vi "ploter.vi"() -> ()   [LabVIEW 2011]
panel:
  in  "SLM 1":bool
  in  "T --> A":bool
  in  "Boolean":bool
  in  "stop":bool
  in  "Quarter Wave Plate":dbl
  in  "Half Wave Plate":dbl
  out "Amplitude":T1(plugin-control)
  out "Phase":T1(plugin-control)
  out "Polar":T1(plugin-control)
  # "SLM 2"
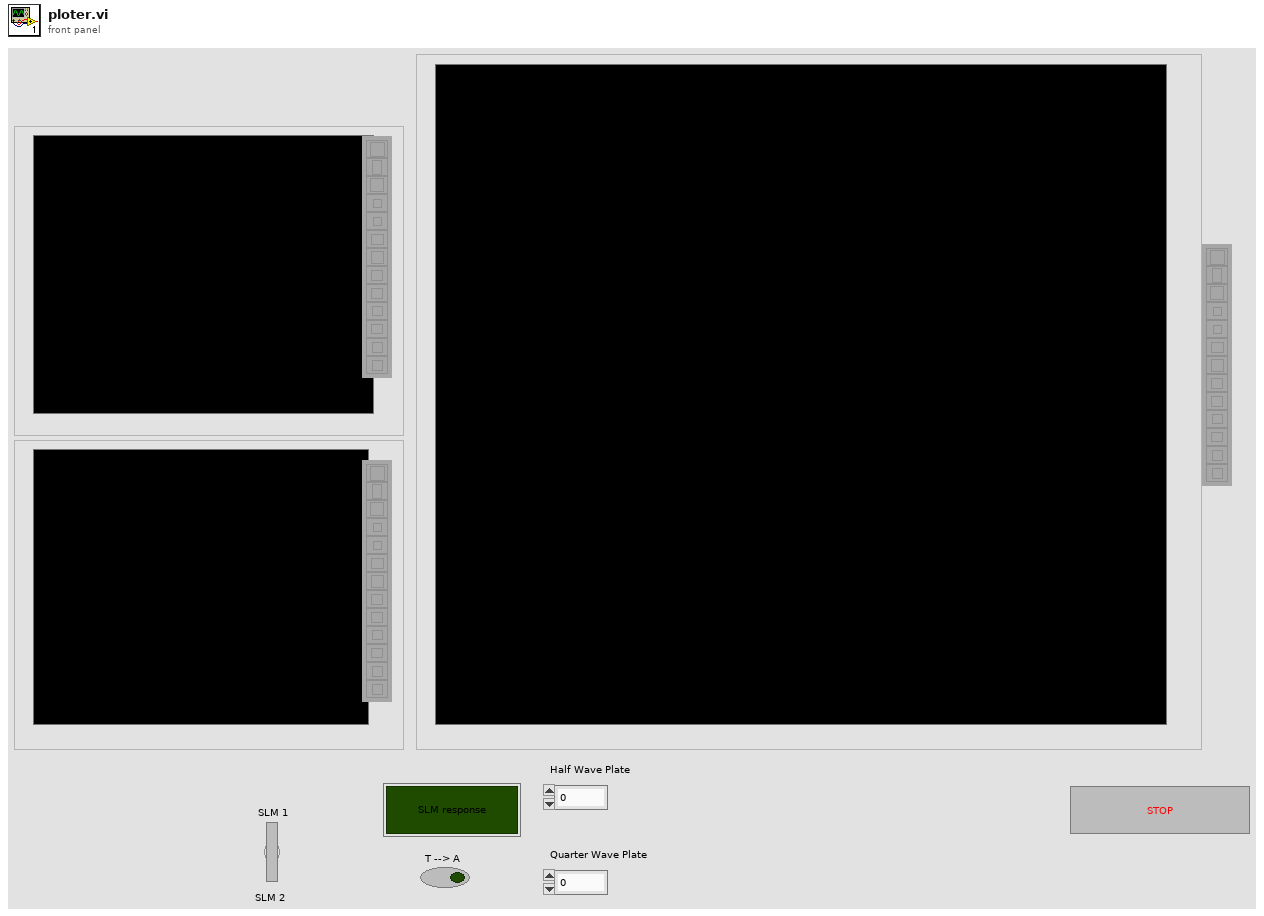
[diagram p1: front panel]
types:
  T1 = typedef "IMAQ Image.ctl" = refnum<image>
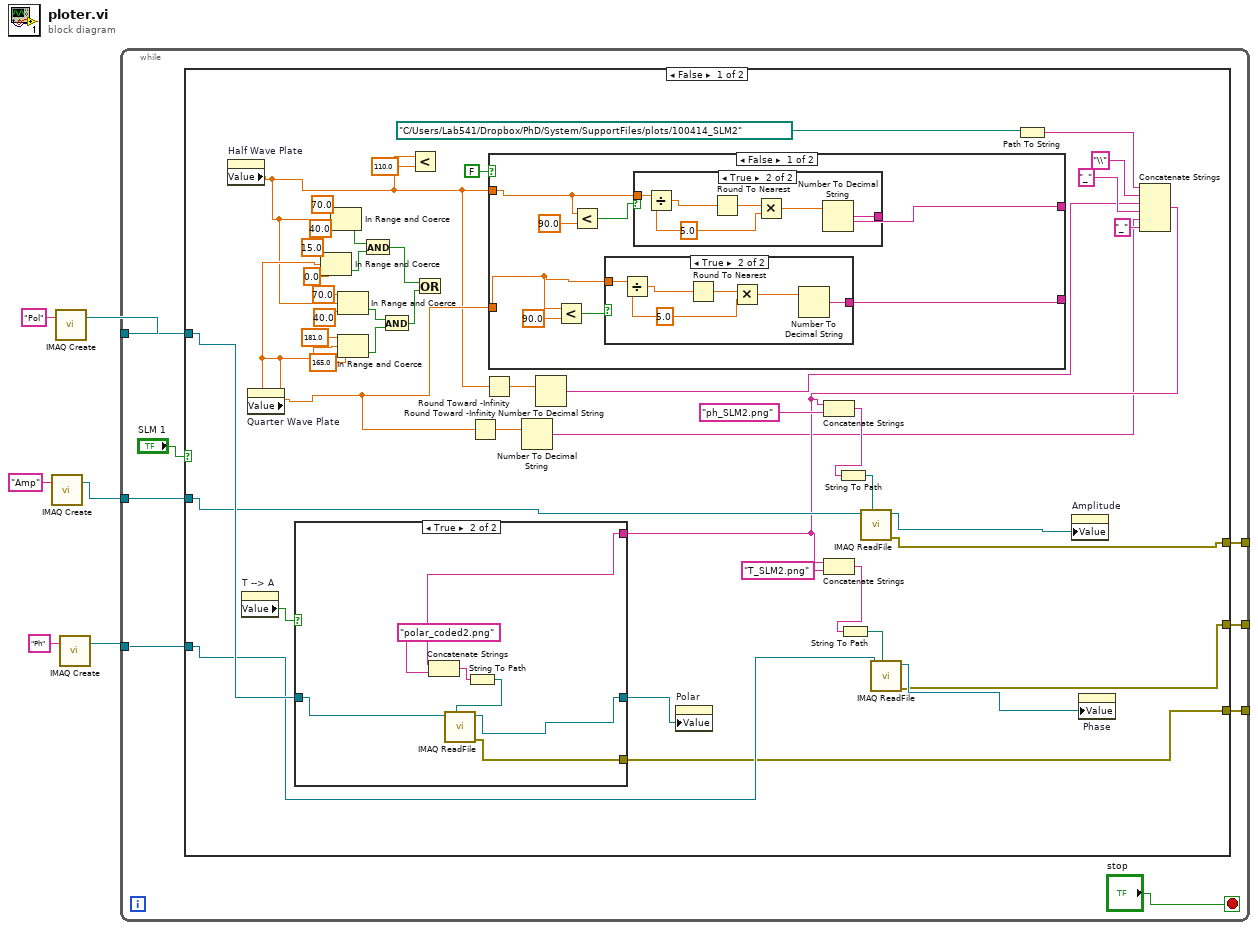
[diagram p0: block diagram]
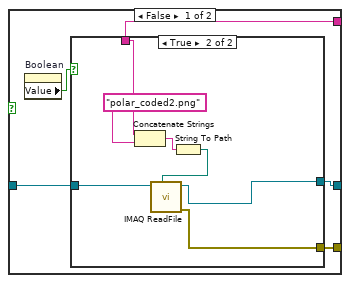
[diagram p2: hidden frame]
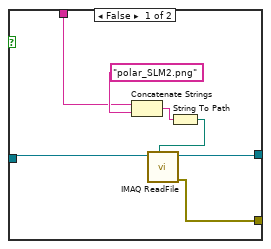
[diagram p3: hidden frame]
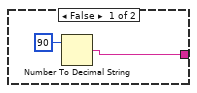
[diagram p4: hidden frame]
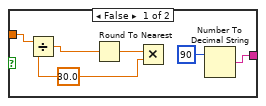
[diagram p5: hidden frame]
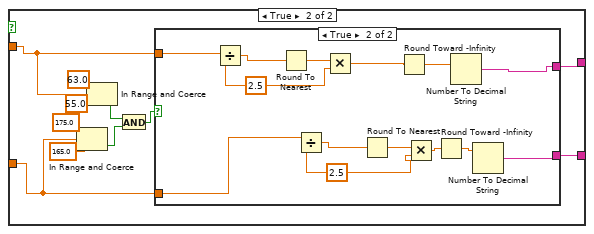
[diagram p6: hidden frame]
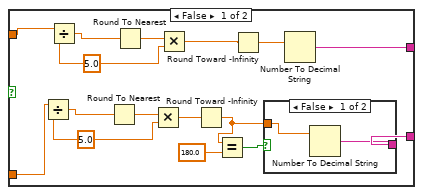
[diagram p7: hidden frame]
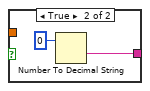
[diagram p8: hidden frame]
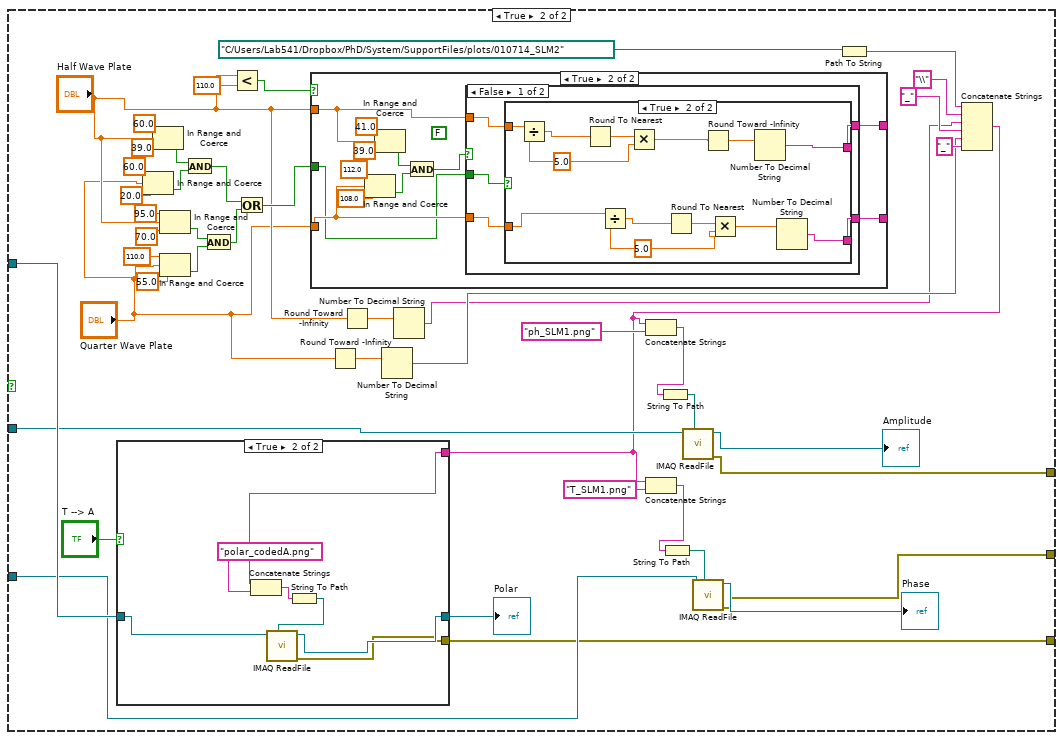
[diagram p9: hidden frame]
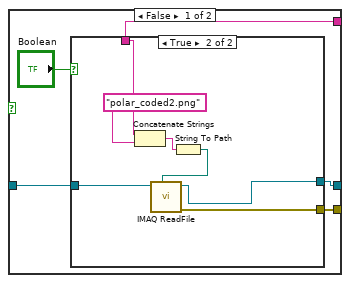
[diagram p10: hidden frame]
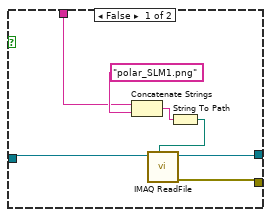
[diagram p11: hidden frame]
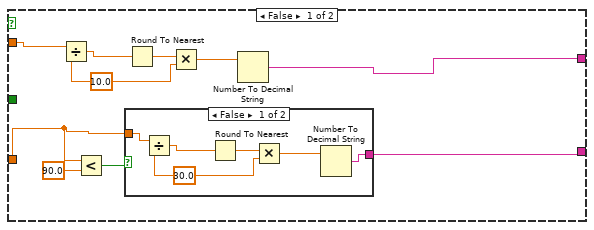
[diagram p12: hidden frame]
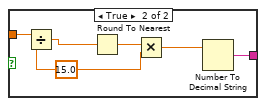
[diagram p13: hidden frame]
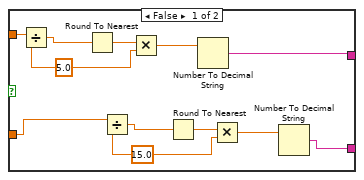
[diagram p14: hidden frame]
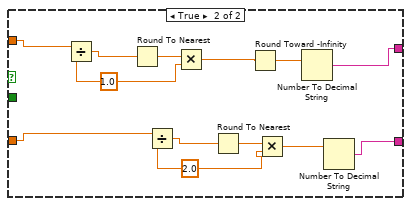
[diagram p15: hidden frame]
diagram:
  n1 = call "IMAQ Create"("Image Name"="Amp") -> ("New Image"=w5:T1)  [unwired: 4 in, 1 out]
  n2 = call "IMAQ Create"("Image Name"="Pol") -> ("New Image"=w6:T1)  [unwired: 4 in, 1 out]
  n3 = call "IMAQ Create"("Image Name"="Ph") -> ("New Image"=w4:T1)  [unwired: 4 in, 1 out]
  n4 = while {
    tunnel: w6 -> [w14]
    tunnel: w5 -> [w13]
    tunnel: w4 -> [w12]
    tunnel: [w9] -> _
    tunnel: [w8] -> _
    tunnel: [w7] -> _
    stop <- "stop" stop-if-true
    n5 = case shown="False" "SLM 1" {
      tunnel: w14 -> [w58 w202]
      tunnel: w13 -> [w57 w201]
      tunnel: w12 -> [w56 w200]
      tunnel: [w21 w166] -> w9
      tunnel: [w22 w165] -> w8
      tunnel: [w23 w164] -> w7
      frame False {
        n6 = property on="Half Wave Plate" class="DigNum (strict)"() -> ("Value"=w17:dbl)  [unwired: 2 in, 2 out]
        n7 = property on="T --> A" class="Bool (strict)"() -> ("Value"=w26:bool)  [unwired: 2 in, 2 out]
        n8 = property on="Quarter Wave Plate" class="DigNum (strict)"() -> ("Value"=w18:dbl)  [unwired: 2 in, 2 out]
        n9 = In Range and Coerce(upper limit=15.0, x=w18, lower limit=0.0) -> (In Range?=w38:bool)  [unwired: 1 out]
        n10 = In Range and Coerce(upper limit=70.0, x=w17, lower limit=40.0) -> (In Range?=w39:bool)  [unwired: 1 out]
        n11 = In Range and Coerce(upper limit=70.0, x=w17, lower limit=40.0) -> (In Range?=w37:bool)  [unwired: 1 out]
        n12 = In Range and Coerce(upper limit=181.0, x=w18, lower limit=165.0) -> (In Range?=w36:bool)  [unwired: 1 out]
        n13 = And(x=w39, y=w38) -> (x .and. y?=w35:bool)
        n14 = And(x=w37, y=w36) -> (x .and. y?=w25:bool)
        n15 = Less?(x=w17, y=110.0) -> ()  [unwired: 1 out]
        n16 = Or(x=w35, y=w25) -> ()  [unwired: 1 out]
        n17 = Round Toward -Infinity(1:w18) -> (0:w19:dbl)
        n18 = Round Toward -Infinity(1:w17) -> (0:w20:dbl)
        n19 = case shown="False" FALSE {
          tunnel: [w92 w123] -> _
          tunnel: [w91 w122] -> _
          tunnel: w18 -> [w90 w114]
          tunnel: w17 -> [w87 w115]
          frame False {
            n20 = Less?(x=w90, y=90.0) -> (x < y?=w88:bool)
            n21 = Less?(x=w87, y=90.0) -> (x < y?=w85:bool)
            n22 = case shown="True" w88 {
              tunnel: w90 -> [w104 w109]
              tunnel: [w103 w108] -> w91
              frame False {
                w102 = 30.0 ("y")
                n23 = Divide(x=w104, y=w102) -> (x/y=w106:dbl)
                n24 = Round To Nearest(number=w106) -> (nearest integer value=w105:dbl)
                n25 = Multiply(x=w105, y=w102) -> ()  [unwired: 1 out]
                n26 = Number To Decimal String(number=90) -> (decimal integer string=w103:string)  [unwired: 1 in]
              }
              frame True {
                w107 = 5.0 ("y")
                n27 = Divide(x=w109, y=w107) -> (x/y=w112:dbl)
                n28 = Round To Nearest(number=w112) -> (nearest integer value=w111:dbl)
                n29 = Multiply(x=w111, y=w107) -> (x*y=w110:dbl)
                n30 = Number To Decimal String(number=w110) -> (decimal integer string=w108:string)  [unwired: 1 in]
              }
            }
            n31 = case shown="True" w85 {
              tunnel: w87 -> [_ w97]
              tunnel: [w94 w96] -> w92
              frame False {
                n32 = Number To Decimal String(number=90) -> (decimal integer string=w94:string)  [unwired: 1 in]
              }
              frame True {
                w95 = 5.0 ("y")
                n33 = Divide(x=w97, y=w95) -> (x/y=w100:dbl)
                n34 = Round To Nearest(number=w100) -> (nearest integer value=w99:dbl)
                n35 = Multiply(x=w99, y=w95) -> (x*y=w98:dbl)
                n36 = Number To Decimal String(number=w98) -> (decimal integer string=w96:string)  [unwired: 1 in]
              }
            }
          }
          frame True {
            n37 = In Range and Coerce(upper limit=175.0, x=w114, lower limit=165.0) -> (In Range?=w116:bool)  [unwired: 1 out]
            n38 = In Range and Coerce(upper limit=63.0, x=w115, lower limit=55.0) -> (In Range?=w117:bool)  [unwired: 1 out]
            n39 = And(x=w117, y=w116) -> (x .and. y?=w113:bool)
            n40 = case shown="True" w113 {
              tunnel: [w130 w147] -> w123
              tunnel: [w129 w146] -> w122
              tunnel: w115 -> [w125 w149]
              tunnel: w114 -> [w124 w148]
              frame False {
                w131 = 5.0 ("y")
                w135 = 5.0 ("y")
                n41 = Divide(x=w124, y=w131) -> (x/y=w134:dbl)
                n42 = Divide(x=w125, y=w135) -> (x/y=w139:dbl)
                n43 = Round To Nearest(number=w134) -> (nearest integer value=w133:dbl)
                n44 = Round To Nearest(number=w139) -> (nearest integer value=w138:dbl)
                n45 = Multiply(x=w133, y=w131) -> (x*y=w132:dbl)
                n46 = Multiply(x=w138, y=w135) -> (x*y=w137:dbl)
                n47 = Round Toward -Infinity(1:w132) -> (0:w128:dbl)
                n48 = Equal?(x=w128, y=180.0) -> (x = y?=w126:bool)
                n49 = Round Toward -Infinity(1:w137) -> (0:w136:dbl)
                n50 = case shown="False" w126 {
                  tunnel: [w140 w143] -> w129
                  tunnel: w128 -> [w141 _]
                  frame False {
                    n51 = Number To Decimal String(number=w141) -> (decimal integer string=w140:string)  [unwired: 1 in]
                  }
                  frame True {
                    n52 = Number To Decimal String(number=0) -> (decimal integer string=w143:string)  [unwired: 1 in]
                  }
                }
                n53 = Number To Decimal String(number=w136) -> (decimal integer string=w130:string)  [unwired: 1 in]
              }
              frame True {
                w150 = 2.5 ("y")
                w151 = 2.5 ("y")
                n54 = Divide(x=w149, y=w151) -> (x/y=w157:dbl)
                n55 = Round To Nearest(number=w157) -> (nearest integer value=w156:dbl)
                n56 = Divide(x=w148, y=w150) -> (x/y=w155:dbl)
                n57 = Multiply(x=w156, y=w151) -> (x*y=w153:dbl)
                n58 = Round To Nearest(number=w155) -> (nearest integer value=w154:dbl)
                n59 = Round Toward -Infinity(1:w153) -> (0:w152:dbl)
                n60 = Multiply(x=w154, y=w150) -> (x*y=w145:dbl)
                n61 = Round Toward -Infinity(1:w145) -> (0:w144:dbl)
                n62 = Number To Decimal String(number=w152) -> (decimal integer string=w147:string)  [unwired: 1 in]
                n63 = Number To Decimal String(number=w144) -> (decimal integer string=w146:string)  [unwired: 1 in]
              }
            }
          }
        }
        n64 = Number To Decimal String(number=w19) -> (decimal integer string=w15:string)  [unwired: 1 in]
        n65 = Number To Decimal String(number=w20) -> (decimal integer string=w16:string)  [unwired: 1 in]
        n66 = Path To String(path=path "C:/Users/Lab541/Dropbox/PhD/System/SupportFiles/plots/100414_SLM2" ("File Path")) -> (string=w52:string)
        n67 = Concatenate Strings(w52, "\\" ("string"), w16, "_" ("string"), w15, "_" ("string")) -> (w41:string)
        n68 = case shown="True" w26 {
          tunnel: w58 -> [w63 w79]
          tunnel: [w62 w80] -> w27
          tunnel: w41 -> [w61 w81]
          tunnel: [w59 w78] -> w21
          frame False {
            n69 = property on="Boolean" class="Bool (strict)"() -> ("Value"=w60:bool)  [unwired: 2 in, 2 out]
            n70 = case shown="True" w60 {
              tunnel: w63 -> [w67 w77]
              tunnel: w61 -> [w65 w73]
              tunnel: [w66 w72] -> w62
              tunnel: [w64 w71] -> w59
              frame False {
                n71 = Concatenate Strings(w65, "polar_SLM2.png" ("string")) -> (w69:string)
                n72 = String To Path(string=w69) -> (path=w68:path)
                n73 = call "IMAQ ReadFile"("File Path"=w68, "Image"=w67) -> ("error out"=w64:errorcluster, "Image Out"=w66:T1)  [unwired: 5 in, 3 out]
              }
              frame True {
                n74 = Concatenate Strings(w73, "polar_coded2.png" ("string")) -> (w75:string)
                n75 = String To Path(string=w75) -> (path=w74:path)
                n76 = call "IMAQ ReadFile"("File Path"=w74, "Image"=w77) -> ("error out"=w71:errorcluster, "Image Out"=w72:T1)  [unwired: 5 in, 3 out]
              }
            }
          }
          frame True {
            n77 = Concatenate Strings(w81, "polar_coded2.png" ("string")) -> (w83:string)
            n78 = String To Path(string=w83) -> (path=w82:path)
            n79 = call "IMAQ ReadFile"("File Path"=w82, "Image"=w79) -> ("error out"=w78:errorcluster, "Image Out"=w80:T1)  [unwired: 5 in, 3 out]
          }
        }
        n80 = property on="Polar" class="ImageControl"("Value"=w27) -> ()  [unwired: 2 in, 2 out]
        n81 = Concatenate Strings(w41, "ph_SLM2.png" ("string")) -> (w49:string)
        n82 = Concatenate Strings(w41, "T_SLM2.png" ("string")) -> (w46:string)
        n83 = String To Path(string=w49) -> (path=w48:path)
        n84 = String To Path(string=w46) -> (path=w45:path)
        n85 = call "IMAQ ReadFile"("File Path"=w48, "Image"=w57) -> ("error out"=w23:errorcluster, "Image Out"=w29:T1)  [unwired: 5 in, 3 out]
        n86 = call "IMAQ ReadFile"("File Path"=w45, "Image"=w56) -> ("error out"=w22:errorcluster, "Image Out"=w28:T1)  [unwired: 5 in, 3 out]
        n87 = property on="Amplitude" class="ImageControl"("Value"=w29) -> ()  [unwired: 2 in, 2 out]
        n88 = property on="Phase" class="ImageControl"("Value"=w28) -> ()  [unwired: 2 in, 2 out]
      }
      frame True {
        n89 = In Range and Coerce(upper limit=60.0, x="Quarter Wave Plate", lower limit=20.0) -> (In Range?=w179:bool)  [unwired: 1 out]
        n90 = In Range and Coerce(upper limit=60.0, x="Half Wave Plate", lower limit=39.0) -> (In Range?=w180:bool)  [unwired: 1 out]
        n91 = In Range and Coerce(upper limit=95.0, x="Half Wave Plate", lower limit=70.0) -> (In Range?=w178:bool)  [unwired: 1 out]
        n92 = In Range and Coerce(upper limit=110.0, x="Quarter Wave Plate", lower limit=55.0) -> (In Range?=w177:bool)  [unwired: 1 out]
        n93 = And(x=w180, y=w179) -> (x .and. y?=w175:bool)
        n94 = And(x=w178, y=w177) -> (x .and. y?=w176:bool)
        n95 = Less?(x="Half Wave Plate", y=110.0) -> (x < y?=w168:bool)
        n96 = Or(x=w175, y=w176) -> (x .or. y?=w174:bool)
        n97 = case shown="True" w168 {
          tunnel: [w234 w262] -> _
          tunnel: [w233 w261] -> _
          tunnel: w174 -> [_ w252]
          tunnel: "Quarter Wave Plate" -> [w232 w253]
          tunnel: "Half Wave Plate" -> [w235 w254]
          frame False {
            w229 = 10.0 ("y")
            n98 = Divide(x=w235, y=w229) -> (x/y=w238:dbl)
            n99 = Less?(x=w232, y=90.0) -> (x < y?=w230:bool)
            n100 = case shown="False" w230 {
              tunnel: w232 -> [w241 w247]
              tunnel: [w240 w246] -> w233
              frame False {
                w239 = 30.0 ("y")
                n101 = Divide(x=w241, y=w239) -> (x/y=w244:dbl)
                n102 = Round To Nearest(number=w244) -> (nearest integer value=w243:dbl)
                n103 = Multiply(x=w243, y=w239) -> (x*y=w242:dbl)
                n104 = Number To Decimal String(number=w242) -> (decimal integer string=w240:string)  [unwired: 1 in]
              }
              frame True {
                w245 = 15.0 ("y")
                n105 = Divide(x=w247, y=w245) -> (x/y=w250:dbl)
                n106 = Round To Nearest(number=w250) -> (nearest integer value=w249:dbl)
                n107 = Multiply(x=w249, y=w245) -> (x*y=w248:dbl)
                n108 = Number To Decimal String(number=w248) -> (decimal integer string=w246:string)  [unwired: 1 in]
              }
            }
            n109 = Round To Nearest(number=w238) -> (nearest integer value=w237:dbl)
            n110 = Multiply(x=w237, y=w229) -> (x*y=w236:dbl)
            n111 = Number To Decimal String(number=w236) -> (decimal integer string=w234:string)  [unwired: 1 in]
          }
          frame True {
            (unwired) FALSE
            n112 = In Range and Coerce(upper limit=112.0, x=w253, lower limit=108.0) -> (In Range?=w255:bool)  [unwired: 1 out]
            n113 = In Range and Coerce(upper limit=41.0, x=w254, lower limit=39.0) -> (In Range?=w256:bool)  [unwired: 1 out]
            n114 = And(x=w256, y=w255) -> (x .and. y?=w251:bool)
            n115 = case shown="False" w251 {
              tunnel: [w267 w294] -> w262
              tunnel: [w266 w293] -> w261
              tunnel: w252 -> [w265 _]
              tunnel: w253 -> [w264 w295]
              tunnel: w254 -> [w263 w296]
              frame False {
                n116 = case shown="True" w265 {
                  tunnel: [w271 w292] -> w267
                  tunnel: [w270 w291] -> w266
                  tunnel: w264 -> [w273 w290]
                  tunnel: w263 -> [w272 w289]
                  frame False {
                    w268 = 15.0 ("y")
                    w269 = 5.0 ("y")
                    n117 = Divide(x=w272, y=w269) -> (x/y=w279:dbl)
                    n118 = Round To Nearest(number=w279) -> (nearest integer value=w278:dbl)
                    n119 = Divide(x=w273, y=w268) -> (x/y=w276:dbl)
                    n120 = Multiply(x=w278, y=w269) -> (x*y=w277:dbl)
                    n121 = Round To Nearest(number=w276) -> (nearest integer value=w275:dbl)
                    n122 = Number To Decimal String(number=w277) -> (decimal integer string=w271:string)  [unwired: 1 in]
                    n123 = Multiply(x=w275, y=w268) -> (x*y=w274:dbl)
                    n124 = Number To Decimal String(number=w274) -> (decimal integer string=w270:string)  [unwired: 1 in]
                  }
                  frame True {
                    w280 = 5.0 ("y")
                    w281 = 5.0 ("y")
                    n125 = Divide(x=w289, y=w281) -> (x/y=w288:dbl)
                    n126 = Round To Nearest(number=w288) -> (nearest integer value=w287:dbl)
                    n127 = Divide(x=w290, y=w280) -> (x/y=w286:dbl)
                    n128 = Multiply(x=w287, y=w281) -> (x*y=w283:dbl)
                    n129 = Round To Nearest(number=w286) -> (nearest integer value=w285:dbl)
                    n130 = Round Toward -Infinity(1:w283) -> (0:w282:dbl)
                    n131 = Multiply(x=w285, y=w280) -> (x*y=w284:dbl)
                    n132 = Number To Decimal String(number=w282) -> (decimal integer string=w292:string)  [unwired: 1 in]
                    n133 = Number To Decimal String(number=w284) -> (decimal integer string=w291:string)  [unwired: 1 in]
                  }
                }
              }
              frame True {
                w297 = 2.0 ("y")
                w298 = 1.0 ("y")
                n134 = Divide(x=w296, y=w298) -> (x/y=w305:dbl)
                n135 = Round To Nearest(number=w305) -> (nearest integer value=w304:dbl)
                n136 = Divide(x=w295, y=w297) -> (x/y=w303:dbl)
                n137 = Multiply(x=w304, y=w298) -> (x*y=w300:dbl)
                n138 = Round To Nearest(number=w303) -> (nearest integer value=w302:dbl)
                n139 = Round Toward -Infinity(1:w300) -> (0:w299:dbl)
                n140 = Multiply(x=w302, y=w297) -> (x*y=w301:dbl)
                n141 = Number To Decimal String(number=w299) -> (decimal integer string=w294:string)  [unwired: 1 in]
                n142 = Number To Decimal String(number=w301) -> (decimal integer string=w293:string)  [unwired: 1 in]
              }
            }
          }
        }
        n143 = Round Toward -Infinity(1:"Quarter Wave Plate") -> (0:w160:dbl)
        n144 = Round Toward -Infinity(1:"Half Wave Plate") -> (0:w161:dbl)
        n145 = Number To Decimal String(number=w160) -> (decimal integer string=w159:string)  [unwired: 1 in]
        n146 = Number To Decimal String(number=w161) -> (decimal integer string=w158:string)  [unwired: 1 in]
        n147 = Path To String(path=path "C:/Users/Lab541/Dropbox/PhD/System/SupportFiles/plots/010714_SLM2" ("File Path")) -> (string=w194:string)
        n148 = Concatenate Strings(w194, "\\" ("string"), w158, "_" ("string"), w159, "_" ("string")) -> (w182:string)
        n149 = case shown="True" "T --> A" {
          tunnel: w202 -> [w207 w223]
          tunnel: [w205 w224] -> w183
          tunnel: w182 -> [w204 w225]
          tunnel: [w203 w222] -> w166
          frame False {
            n150 = case shown="True" "Boolean" {
              tunnel: w207 -> [w211 w221]
              tunnel: w204 -> [w209 w217]
              tunnel: [w210 w216] -> w205
              tunnel: [w208 w215] -> w203
              frame False {
                n151 = Concatenate Strings(w209, "polar_SLM1.png" ("string")) -> (w213:string)
                n152 = String To Path(string=w213) -> (path=w212:path)
                n153 = call "IMAQ ReadFile"("File Path"=w212, "Image"=w211) -> ("error out"=w208:errorcluster, "Image Out"=w210:T1)  [unwired: 5 in, 3 out]
              }
              frame True {
                n154 = Concatenate Strings(w217, "polar_coded2.png" ("string")) -> (w219:string)
                n155 = String To Path(string=w219) -> (path=w218:path)
                n156 = call "IMAQ ReadFile"("File Path"=w218, "Image"=w221) -> ("error out"=w215:errorcluster, "Image Out"=w216:T1)  [unwired: 5 in, 3 out]
              }
            }
          }
          frame True {
            n157 = Concatenate Strings(w225, "polar_codedA.png" ("string")) -> (w227:string)
            n158 = String To Path(string=w227) -> (path=w226:path)
            n159 = call "IMAQ ReadFile"("File Path"=w226, "Image"=w223) -> ("error out"=w222:errorcluster, "Image Out"=w224:T1)  [unwired: 5 in, 3 out]
          }
        }
        "Polar" <- w183
        n160 = Concatenate Strings(w182, "ph_SLM1.png" ("string")) -> (w191:string)
        n161 = Concatenate Strings(w182, "T_SLM1.png" ("string")) -> (w188:string)
        n162 = String To Path(string=w191) -> (path=w190:path)
        n163 = String To Path(string=w188) -> (path=w187:path)
        n164 = call "IMAQ ReadFile"("File Path"=w190, "Image"=w201) -> ("error out"=w164:errorcluster, "Image Out"=→"Amplitude":T1)  [unwired: 5 in, 3 out]
        n165 = call "IMAQ ReadFile"("File Path"=w187, "Image"=w200) -> ("error out"=w165:errorcluster, "Image Out"=→"Phase":T1)  [unwired: 5 in, 3 out]
      }
    }
  }
